vi "Xeryon build statusbits array.vi"(3 "Array in":T2(array[cluster])) -> (1 "Array":T3[](array[typedef]))   [LabVIEW 2019]
uses:
  Xeryon status bits.ctl
  Serial driver/Serial parameters.ctl
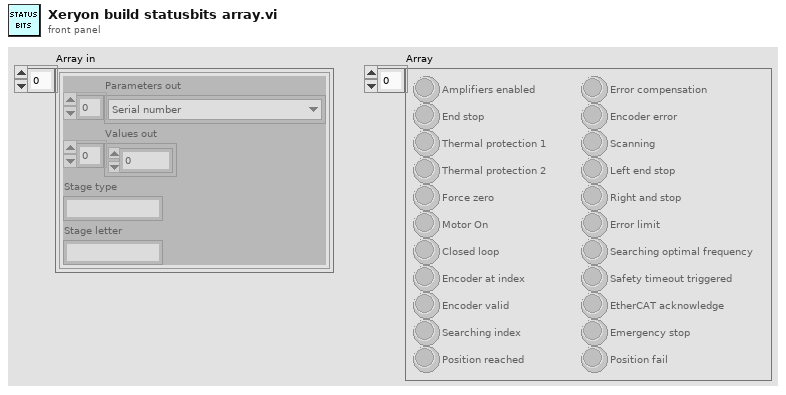
[diagram p1: front panel]
types:
  T1 = typedef "Serial parameters.ctl" = enum16{"Serial number", "Software number", "Type of stage", "Status", "Frequency", "Encoder position", "Desired position", "Info", "Phase correction", "Timestamp", "Proportional control factor", "Sync", "XRT1", "XRT3", "XRTA", "XLS1", "XLS3", "XLA1", "XLA3"}
  T2 = cluster{"Parameters out":T1[], "Values out":i32[], "Stage type":string, "Stage letter":string}[]
  T3 = typedef "Xeryon status bits.ctl" = cluster{"Amplifiers enabled":bool, "End stop":bool, "Thermal protection 1":bool, "Thermal protection 2":bool, "Force zero":bool, "Motor On":bool, "Closed loop":bool, "Encoder at index":bool, "Encoder valid":bool, "Searching index":bool, "Position reached":bool, "Error compensation":bool, "Encoder error":bool, "Scanning":bool, "Left end stop":bool, "Right and stop":bool, "Error limit":bool, "Searching optimal frequency":bool, "Safety timeout triggered":bool, "EtherCAT acknowledge":bool, "Emergency stop":bool, "Position fail":bool}
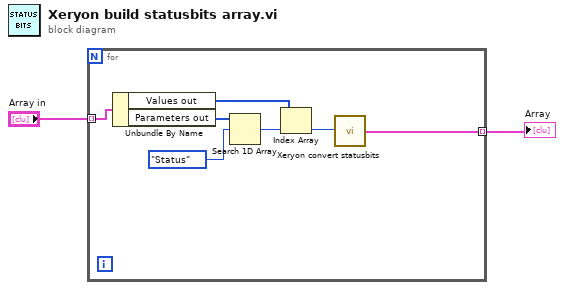
[diagram p0: block diagram]
diagram:
  n1 = for {
    tunnel: "Array in" -> [w9] mode=indexing
    tunnel: [w3] -> w2 mode=indexing
    n2 = Unbundle By Name(w9) -> ("Values out"=w6:i32[], "Parameters out"=w8:T1[])
    n3 = Search 1D Array(1D array=w8, element=Serial_parameters."Status") -> (index of element=w5:i32)  [unwired: 1 in]
    n4 = Index Array(array=w6, index=w5) -> (element=w4:i32)
    n5 = call "Xeryon convert statusbits.vi"("single value out"=w4) -> ("Cluster"=w3:T3)  [unwired: 4 in]
  }
  "Array" <- w2
